vi "Write new data number Msg.vi"(10 "TouchScreen.lvlib:new data number Msg.lvclass":refnum<class "new data number Msg.lvclass">, 11 "TouchScreen in":refnum<class "TouchScreen.lvclass">) -> (3 "TouchScreen out":refnum<class "TouchScreen.lvclass">)   [LabVIEW 2020, in "TouchScreen.lvlib" / "TouchScreen.lvclass"]
uses:
  TouchScreen.lvclass
  TouchScreen Messages/new data number Msg/new data number Msg.lvclass
  TouchScreen.lvclass/TouchScreen.ctl
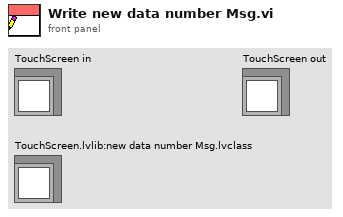
[diagram p1: front panel]
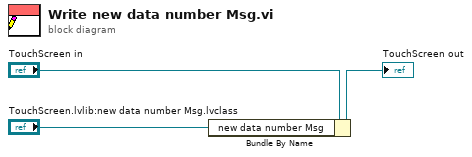
[diagram p0: block diagram]
diagram:
  n1 = Bundle By Name(cluster="TouchScreen in", "new data number Msg"="TouchScreen.lvlib:new data number Msg.lvclass") -> (→"TouchScreen out":refnum<class "TouchScreen.lvclass">)
